vi "AngleIntensitySweep.vi"(8 "error in (no error)":errorcluster, 9 "Rf":dbl, 10 "Num Points":i32, 11 "LINX Resource":T1) -> (0 "Error Out":errorcluster, 1 "PD Current (A)":dbl[](array[numeric]), 2 "Angle":dbl[](array[numeric]), 3 "LINX Resource 2":T1)   [LabVIEW 2020]
uses:
  <vilib>/MakerHub/LINX/Private/Type Defs/LINX Ref.ctl
  <vilib>/MakerHub/LINX/Private/Type Defs/Platform.ctl
  <vilib>/MakerHub/LINX/Private/Type Defs/Interface.ctl
  <vilib>/MakerHub/LINX/Private/Device/Type Defs/LINX Device Config.ctl
  <vilib>/MakerHub/LINX/Private/Device/Type Defs/TCP Config.ctl
  <vilib>/MakerHub/LINX/Private/Device/Type Defs/Channels.ctl
  <vilib>/MakerHub/LINX/LMH-LINX.lvlib
  <vilib>/MakerHub/LINX/Private/Device/Device.lvlib
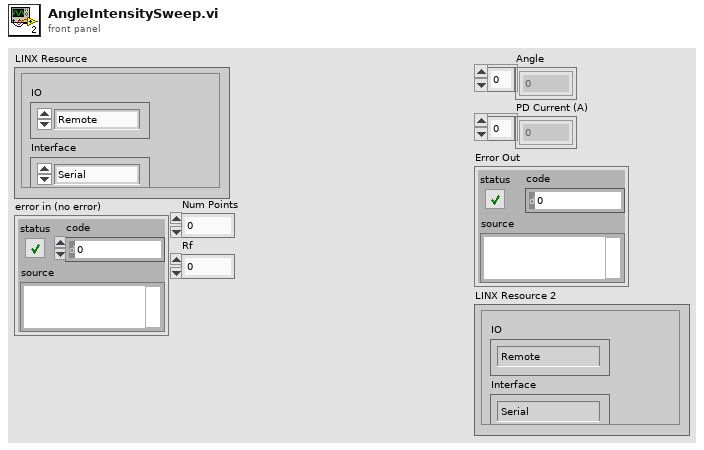
[diagram p1: front panel]
types:
  T1 = typedef "LMH-LINX.lvlib/LINX Ref.ctl" = cluster{"IO":T2, "Interface":T3, "LINX Device Config":T4}
  T2 = typedef "LMH-LINX.lvlib/Platform.ctl" = enum16{"Remote", "Local"}
  T3 = typedef "LMH-LINX.lvlib/Interface.ctl" = enum16{"Serial", "TCP"}
  T4 = typedef "LMH-LINX.lvlib/Device.lvlib/LINX Device Config.ctl" = cluster{"Interface":T3, "COM Port":refnum<visa-resource-name>, "TCP Configuration":T5, "Device Family":u8, "Device ID":u8, "Device Name":string, "TCP Ref":refnum<k5>, "Channels":T6}
  T5 = typedef "LMH-LINX.lvlib/Device.lvlib/TCP Config.ctl" = cluster{"IP Address":string, "Port":u16}
  T6 = typedef "LMH-LINX.lvlib/Channels.ctl" = cluster{"DI":u8[], "DO":u8[], "AI":u8[], "AO":u8[], "PWM":u8[], "QE":u8[], "UART":u8[], "I2C 2":u8[], "SPI":u8[], "CAN":u8[], "Servo":u8[], "AI Ref (V)":dbl, "AI Resolution (Bits)":u8, "AO Ref (V)":dbl, "AO Resolution (Bits)":u8}
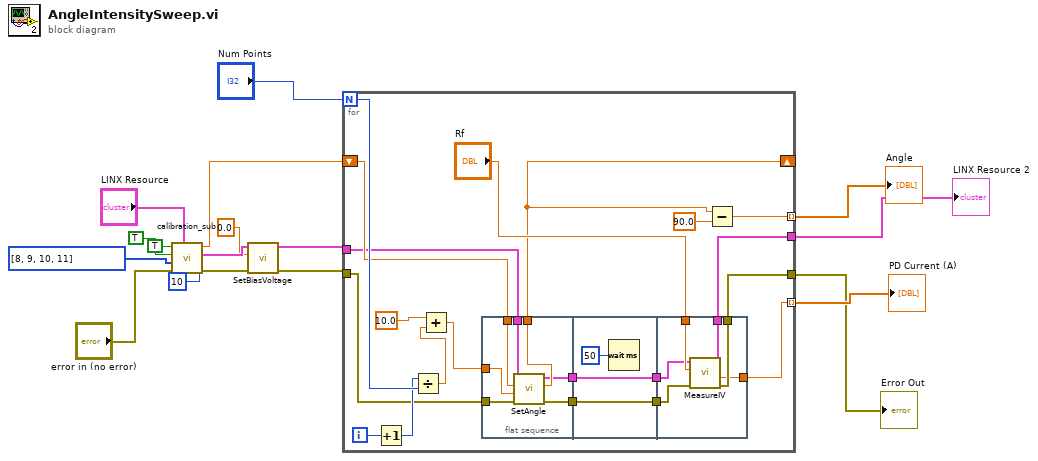
[diagram p0: block diagram]
diagram:
  n1 = call "calibration_sub.vi"("Angle in"=10, "LINX Resource"="LINX Resource", "error in (no error)"="error in (no error)", "DO Channels"=u8[] [8, 9, 10, 11], "CCW"=TRUE, "Start calibration"=TRUE) -> ("error out"=w8:errorcluster, "LINX Resource out"=w9:T1, "Actual angle out"=w11:dbl)  [unwired: 3 in]
  n2 = call "SetBiasVoltage.vi"("Error In"=w8, "Bias V"=0.0, "LINX Resource"=w9) -> ("Error Out"=w5:errorcluster, "LINX Resource 2"=w6:T1)  [unwired: 5 in]
  n3 = for {
    N: "Num Points" -> [w36]
    tunnel: w5 -> [w26]
    tunnel: w6 -> [w23]
    shift-right: [w22] -> _
    shift-left: w11 -> [w24]
    tunnel: [w27] -> w1
    tunnel: [w29] -> w2
    tunnel: [w28] -> w3 mode=indexing
    tunnel: [w32] -> w4 mode=indexing
    i -> [w33]
    n4 = Increment(x=w33) -> (x+1=w34:i32)
    n5 = Divide(x=w34, y=w36) -> (x/y=w35:dbl)
    n6 = Add(x=10.0, y=w35) -> (x+y=w25:dbl)
    n7 = flat-sequence {
      tunnel: w26 -> [w44]
      tunnel: w25 -> [w43]
      tunnel: w24 -> [w42]
      tunnel: w23 -> [w41]
      tunnel: [w40] -> w22
      tunnel: [w39] -> w21
      tunnel: [w38] -> w19
      tunnel: w21 -> [w47]
      tunnel: [w47] -> w20
      tunnel: w19 -> [w46]
      tunnel: [w46] -> w18
      tunnel: "Rf" -> [w53]
      tunnel: [w52] -> w29
      tunnel: [w51] -> w28
      tunnel: [w50] -> w27
      tunnel: w20 -> [w49]
      tunnel: w18 -> [w48]
      frame #0 {
        n8 = call "SetAngle.vi"("error in (no error)"=w44, "TargetAngle"=w43, "Start Angle"=w42, "LINX Resource in"=w41) -> ("error out"=w39:errorcluster, "OutAngle"=w40:dbl, "LINX Resource out"=w38:T1)  [unwired: 5 in]
      }
      frame #1 {
        n9 = Wait (ms)(milliseconds to wait=u32 50) -> ()  [unwired: 1 out]
      }
      frame #2 {
        n10 = call "MeasureIV.vi"("Error In"=w49, "Rf"=w53, "LINX Resource"=w48) -> ("Error Out"=w52:errorcluster, "PD Current (A)"=w51:dbl, "LINX Resource 2"=w50:T1)  [unwired: 5 in, 1 out]
      }
    }
    n11 = Subtract(x=w22, y=90.0) -> (x-y=w32:dbl)
  }
  "Angle" <- w4
  "PD Current (A)" <- w3
  "Error Out" <- w2
  "LINX Resource 2" <- w1
